vi "Check Amplitude Offset Bounds.vi"(6 "MinV":dbl, 7 "Last Iter In Bounds?":bool, 9 "MaxV":dbl, 10 "Offset":dbl, 11 "Amplitude":dbl) -> (1 "Coerced Offset":dbl, 2 "Values In Bounds?":bool, 3 "Coerced Amplitude":dbl)   [LabVIEW 2020, in "Waveform Analog Output Engine.lvlib"]
uses:
  Waveform Analog Output Engine.lvlib
  Console Message Type.ctl
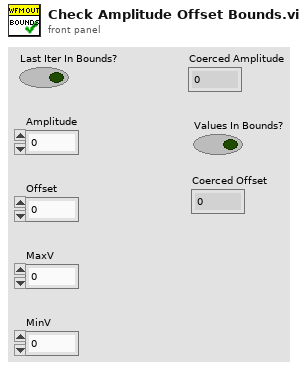
[diagram p1: front panel]
types:
  T1 = typedef "Waveform Analog Output Engine.lvlib/Console Message Type.ctl" = enum16{"Range Warning", "Error"}
  T2 = cluster{"Hw Max":dbl, "Hw Min":dbl, "Requested Amplitude":dbl, "Requested Offset":dbl, "Coerced Amplitude":dbl, "Coerced Offset":dbl}
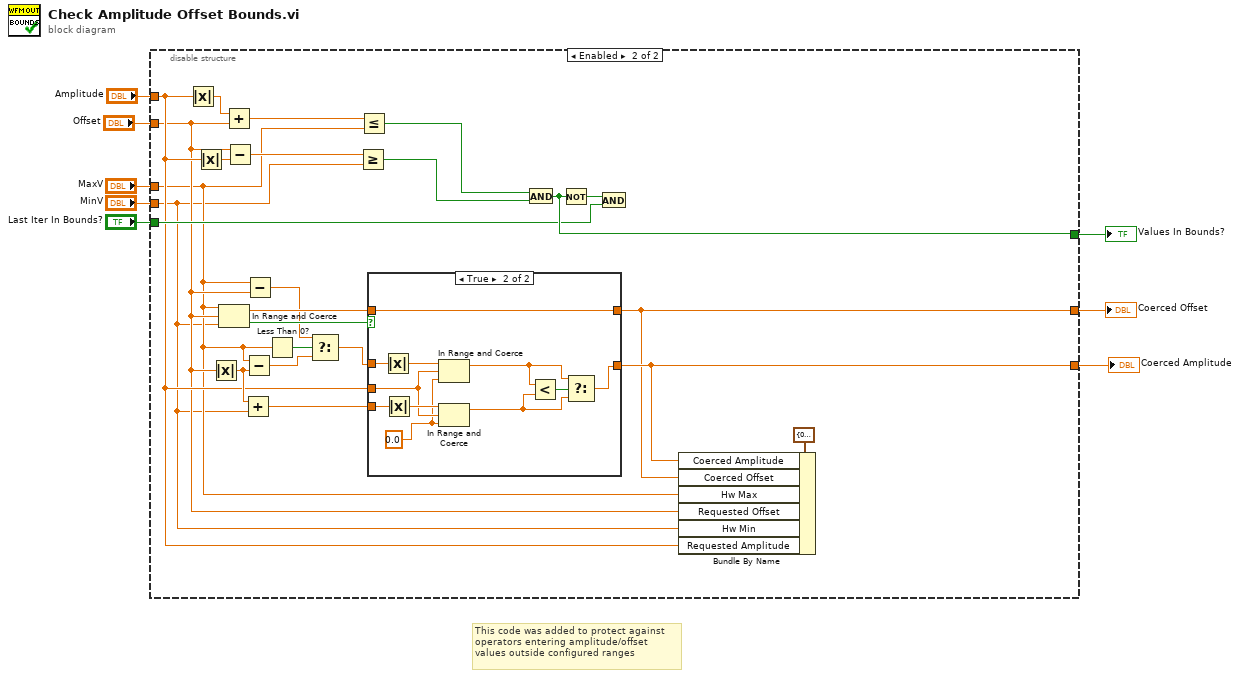
[diagram p0: block diagram]
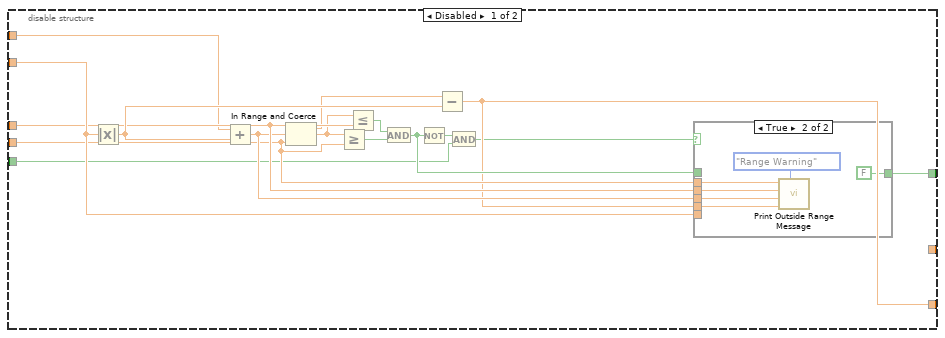
[diagram p2: hidden frame]
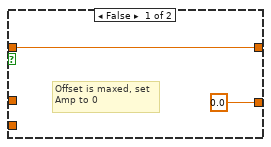
[diagram p4: hidden frame]
diagram:
  # "This code was added to protect against\noperators entering amplitude/offset\nvalues outside configured ranges"
  n1 = disable-structure shown="Enabled" {
    disable-tunnel: "Offset" -> [w23 w34]
    disable-tunnel: "MaxV" -> [w18 w33]
    disable-tunnel: "MinV" -> [w16 w32]
    disable-tunnel: [w15 w37] -> w5
    disable-tunnel: "Amplitude" -> [w13 w42]
    disable-tunnel: [w12 w55] -> w3
    disable-tunnel: "Last Iter In Bounds?" -> [w10 w54]
    disable-tunnel: [_ w36] -> w1
    frame Disabled {
      n2 = Absolute Value(x=w23) -> (abs(x)=w22:dbl)
      n3 = Add(x=w13, y=w22) -> (x+y=w17:dbl)
      n4 = In Range and Coerce(upper limit=w18, x=w17, lower limit=w16) -> (coerced(x)=w14:dbl)  [unwired: 1 out]
      n5 = Greater Or Equal?(x=w17, y=w16) -> (x >= y?=w20:bool)
      n6 = Less Or Equal?(x=w17, y=w18) -> (x <= y?=w19:bool)
      n7 = And(x=w19, y=w20) -> (x .and. y?=w21:bool)
      n8 = Not(x=w21) -> (.not. x?=w9:bool)
      n9 = Subtract(x=w14, y=w22) -> (x-y=w15:dbl)
      n10 = And(x=w9, y=w10) -> (x .and. y?=w11:bool)
      n11 = case shown="True" w11 {
        tunnel: w16 -> [_ w31]
        tunnel: w18 -> [_ w30]
        tunnel: w17 -> [_ w29]
        tunnel: w15 -> [_ w28]
        tunnel: w21 -> [w24 _]
        tunnel: [w24 FALSE] -> w12
        tunnel: w23 -> [_ w25]
        frame False {
        }
        frame True {
          n12 = call "Print Outside Range Message.vi"(4:w25, 6:w28, "Message Type"=Console_Message_Type."Range Warning", 9:w29, 10:w30, "Message Values"=w31) -> ()  [unwired: 6 in]
        }
      }
    }
    frame Enabled {
      n13 = Absolute Value(x=w42) -> (abs(x)=w35:dbl)
      n14 = Absolute Value(x=w42) -> (abs(x)=w43:dbl)
      n15 = Absolute Value(x=w34) -> (abs(x)=w46:dbl)
      n16 = In Range and Coerce(upper limit=w33, x=w34, lower limit=w32) -> (coerced(x)=w47:dbl, In Range?=w48:bool)
      n17 = Add(x=w35, y=w34) -> (x+y=w52:dbl)
      n18 = Subtract(x=w34, y=w43) -> (x-y=w51:dbl)
      n19 = Add(x=w46, y=w32) -> (x+y=w45:dbl)
      n20 = Subtract(x=w33, y=w46) -> (x-y=w40:dbl)
      n21 = Subtract(x=w33, y=w34) -> (x-y=w39:dbl)
      n22 = Less Than 0?(x=w33) -> (x < 0?=w41:bool)
      n23 = Select(t=w39, s=w41, f=w40) -> (s? t:f=w38:dbl)
      n24 = Greater Or Equal?(x=w51, y=w32) -> (x >= y?=w49:bool)
      n25 = Less Or Equal?(x=w52, y=w33) -> (x <= y?=w50:bool)
      n26 = case shown="True" w48 {
        tunnel: w47 -> [w57 w68]
        tunnel: [w57 w68] -> w36
        tunnel: [0.0 ("Coerced Amplitude") w60] -> w37
        tunnel: w38 -> [_ w67]
        tunnel: w45 -> [_ w66]
        tunnel: w42 -> [_ w63]
        frame False {
          # "Offset is maxed, set\nAmp to 0"
        }
        frame True {
          w62 = 0.0
          n27 = Absolute Value(x=w67) -> (abs(x)=w65:dbl)
          n28 = Absolute Value(x=w66) -> (abs(x)=w64:dbl)
          n29 = In Range and Coerce(upper limit=w65, x=w63, lower limit=w62) -> (coerced(x)=w58:dbl)  [unwired: 1 out]
          n30 = In Range and Coerce(upper limit=w64, x=w63, lower limit=w62) -> (coerced(x)=w59:dbl)  [unwired: 1 out]
          n31 = Less?(x=w58, y=w59) -> (x < y?=w61:bool)
          n32 = Select(t=w58, s=w61, f=w59) -> (s? t:f=w60:dbl)
        }
      }
      n33 = And(x=w50, y=w49) -> (x .and. y?=w55:bool)
      n34 = Not(x=w55) -> (.not. x?=w53:bool)
      n35 = And(x=w53, y=w54) -> ()  [unwired: 1 out]
      n36 = Bundle By Name(cluster=T2 {"Hw Max"=0.0, "Hw Min"=0.0, "Requested Amplitude"=0.0, "Requested Offset"=0.0, "Coerced Amplitude"=0.0, "Coerced Offset"=0.0} ("Message Values"), "Coerced Amplitude"=w37, "Coerced Offset"=w36, "Hw Max"=w33, "Requested Offset"=w34, "Hw Min"=w32, "Requested Amplitude"=w42) -> ()  [unwired: 1 out]
    }
  }
  "Coerced Amplitude" <- w5
  "Values In Bounds?" <- w3
  "Coerced Offset" <- w1
